vi "Teleop.vi"(10 "Match Info":T1={"Autonomous Elapsed Seconds"=0.0, "TeleOp Elapsed Seconds"=0.0, "Disabled Elapsed Seconds"=0.0, "Visited Autonomous"=FALSE, "Visited TeleOp"=FALSE, "Visited Disabled"=FALSE, "Autonomous Settings"={"Autonomous Style"=enum."Independent", "VI Refnum"=refnum}}, 11 "Call Context":T2) -> ()   [LabVIEW 2015]
doc: "This VI is called for each TeleOp packet received from the DS where the robot is not disabled. It is often used to read from the joysticks and update I/O or to update setpoints for timed control loops. It should complete and return within 20 milliseconds or it may miss DS packets."
uses:
  <vilib>/Rock Robotics/WPI/DriverStation/WPI_DriverStationDerivedRobotMode.ctl
  <vilib>/Rock Robotics/WPI/DriverStation/WPI_DriverStationMatch Info.ctl
  <vilib>/Rock Robotics/WPI/Utilities/WPI_GetSetVariantRefNum.vi
  Robot Global Data.vi
  <vilib>/Rock Robotics/Network Tables/SD Write Number.vi
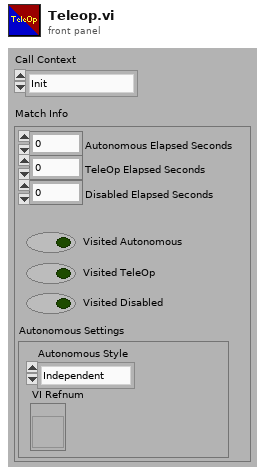
[diagram p1: front panel]
types:
  T1 = typedef "WPI_DriverStationMatch Info.ctl" = cluster{"Autonomous Elapsed Seconds":dbl, "TeleOp Elapsed Seconds":dbl, "Disabled Elapsed Seconds":dbl, "Visited Autonomous":bool, "Visited TeleOp":bool, "Visited Disabled":bool, "Autonomous Settings":cluster{"Autonomous Style":enum16{"Iterative", "Independent"}, "VI Refnum":refnum<vi>}}
  T2 = typedef "WPI_DriverStationDerivedRobotMode.ctl" = enum16{"Init", "Execute", "Stop"}
  T3 = typedef "WPI_RobotDriveDevRef.ctl" = cluster{"DevStatus":errorcluster, "Motors[]":T4[], "Square Inputs":bool, "Max Output":dbl}
  T4 = typedef "WPI_MotorControlDeviceRef.ctl" = cluster{"DeviceStatus":errorcluster, "Type":T5, "PWM":cluster{"PWM Channel":T6, "DeadBand":T7}, "CAN":cluster{"Device Number":u8, "Control Mode":T8, "Semaphore":T9, "Max Vout":dbl, "TalonSRX Control Mode":T10}, "Invert":bool}
  T5 = typedef "WPI_MotorControlType.ctl" = enum16{"PWM", "CAN", "CANTalonSRX"}
  T6 = typedef "FPGA_DIOPWMChannel.ctl" = enum8{"PWM 0", "PWM 1", "PWM 2", "PWM 3", "PWM 4", "PWM 5", "PWM 6", "PWM 7", "PWM 8", "PWM 9", "PWM MXP 0", "PWM MXP 1", "PWM MXP 2", "PWM MXP 3", "PWM MXP 4", "PWM MXP 5", "PWM MXP 6", "PWM MXP 7", "PWM MXP 8", "PWM MXP 9", "Invalid"}
  T7 = typedef "WPI_PWMDeadband.ctl" = cluster{"Name":string, "maxPositivePwm":i32, "minPositivePwm":i32, "centerPwm":i32, "maxNegativePwm":i32, "minNegativePwm":i32, "angularRange":u16}
  T8 = typedef "WPI_CANJaguar_ControlMode.ctl" = enum8{"Percent VBus", "Current", "Speed", "Position", "Voltage"}
  T9 = typedef "Semaphore RefNum" = refnum<k1>
  T10 = typedef "WPI_CANTalonSRX_APIControlMode.ctl" = enum8{"Percent VBus", "Speed", "Position", "Slave", "Unchanged / Invalid", "Voltage Compensation", "Current", "Motion Profile"}
  T11 = typedef "WPI_CANTalonSRX_GlobalStatus.ctl" = cluster{"Applied Throttle":dbl, "Module Enabled":bool, "CAN Error":errorcluster, "Closed Loop Error":dbl, "Forward Limit Switch Closed":bool, "Reverse Limit Switch Closed":bool, "Sensor Position":dbl, "Sensor Velocity":dbl, "Current":dbl, "Sticky Fault - Over Temp":bool, "Sticky Fault - Under Voltage":bool, "Sticky Fault - Forward Limit":bool, "Sticky Fault - Reverse Limit":bool, "Sticky Fault - Forward Soft Limit":bool, "Sticky Fault - Reverse Soft Limit":bool, "Brake is Enabled":bool, "Encoder Position":dbl, "Encoder Velocity":dbl, "Encoder Index Count":dbl, "Encoder A Pin State":bool, "Encoder B Pin State":bool, "Encoder Index Pin State":bool, "Analog In":dbl, "Analog In Velocity":dbl, "Temperature (C)":dbl, "Battery Voltage":dbl, "Control 5 Is Supported":bool, "Current Profile Slot Select":dbl, "Pos Div 8":bool, "Vel Div 4":bool, "Pulse Width Position":i32, "Pulse Width Velocity":i32, "Pulse Width Rise To Rise (us)":i32, "Pulse Width Rise To Fall (us)":i32, "Mot Prof Active Is Under Run":bool, "Mot Prof Active Has Under Run":bool, "Mot Prof Active Is Last":bool, "Mot Prof Active Velocity Only":bool, "Mot Prof Active Is Valid":bool, "Mot Prof Buffer Is Full":bool, "Mot Prof Active Profile Slot Select":i32, "Mot Prof NextID":i32, "Mot Prof Count":i32, "Mot Prof Active Velocity":dbl, "Mot Prof Active Position":dbl, "Mot Prof Output Enable":i32}
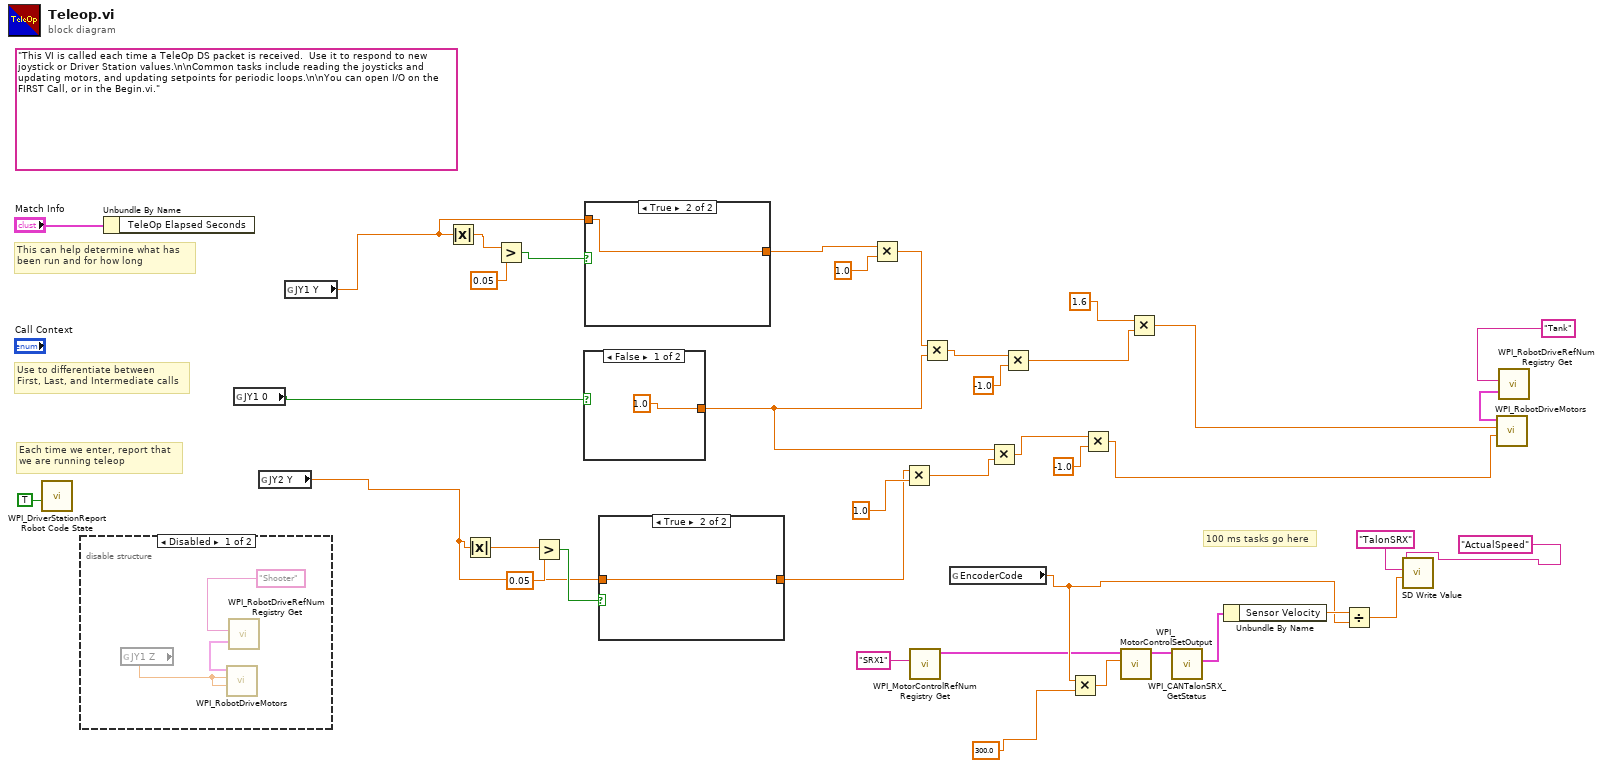
[diagram p0: block diagram]
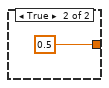
[diagram p3: hidden frame]
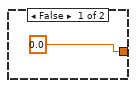
[diagram p4: hidden frame]
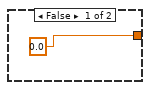
[diagram p5: hidden frame]
diagram:
  (unwired) "This VI is called each time a TeleOp DS packet is received.  Use it to respond to new joystick or Driver Station values.\n\nCommon tasks include reading the joysticks and updating motors, and updating setpoints for periodic loops.\n\nYou can open I/O on the FIRST Call, or in the Begin.vi."
  # "100 ms tasks go here"
  # "Each time we enter, report that\nwe are running teleop"
  # "Use to differentiate between\nFirst, Last, and Intermediate calls"
  # "This can help determine what has\nbeen run and for how long"
  n1 = call <vilib>:"WPI_DriverStationReport Robot Code State.vi"("TeleOp"=TRUE ("Autonomous")) -> ()  [unwired: 10 in, 1 out]
  n2 = disable-structure shown="Disabled" {
    frame Disabled {
      n3 = global read "Robot Global Data.vi" "JY1 Z"() -> (w40:dbl)
      n4 = call <vilib>:"WPI_RobotDriveRefNum Registry Get.vi"("refnum name"="Shooter") -> ("RobotDriveDevRef"=w41:T3)  [unwired: 1 in, 9 out]
      n5 = call <vilib>:"WPI_RobotDriveMotors.vi"("RightSpeed"=w40, "LeftSpeed"=w40, "RobotDriveDevRef"=w41) -> ()  [unwired: 6 in, 3 out]
    }
    frame Enabled {
    }
  }
  n6 = Unbundle By Name("Match Info") -> ()  [unwired: 1 out]
  n7 = global read "Robot Global Data.vi" "JY1 0"() -> (w12:bool)
  n8 = global read "Robot Global Data.vi" "JY2 Y"() -> (w13:dbl)
  n9 = global read "Robot Global Data.vi" "JY1 Y"() -> (w14:dbl)
  n10 = Absolute Value(x=w14) -> (abs(x)=w19:dbl)
  n11 = Absolute Value(x=w13) -> (abs(x)=w18:dbl)
  n12 = Greater?(x=w19, y=0.05) -> (0:w37:bool)
  n13 = Greater?(x=w18, y=0.05) -> (0:w35:bool)
  n14 = case shown="False" w12 {
    tunnel: [1.0 0.5] -> w26
    frame False {
    }
    frame True {
    }
  }
  n15 = case shown="True" w37 {
    tunnel: [0.0 w46] -> w31
    tunnel: w14 -> [_ w46]
    frame False {
    }
    frame True {
    }
  }
  n16 = case shown="True" w35 {
    tunnel: [0.0 w48] -> w30
    tunnel: w13 -> [_ _]
    tunnel: w13 -> [_ w48]
    frame False {
    }
    frame True {
    }
  }
  n17 = Multiply(x=w31, y=1.0) -> (x*y=w27:dbl)
  n18 = Multiply(x=w30, y=1.0) -> (x*y=w25:dbl)
  n19 = call <vilib>:"WPI_MotorControlRefNum Registry Get.vi"("refnum name"="SRX1") -> ("MotorControlDevRef"=w5:T4)  [unwired: 9 in, 1 out]
  n20 = Multiply(x=w27, y=w26) -> (x*y=w24:dbl)
  n21 = global read "Robot Global Data.vi" "EncoderCode"() -> (w7:dbl)
  n22 = Multiply(x=w26, y=w25) -> (x*y=w20:dbl)
  n23 = Multiply(x=w24, y=-1.0) -> (x*y=w16:dbl)
  n24 = Multiply(x=w7, y=300.0) -> (x*y=w8:dbl)
  n25 = Multiply(x=w20, y=-1.0) -> (x*y=w21:dbl)
  n26 = call <vilib>:"WPI_MotorControlSetOutput.vi"("Output"=w8, "MotorControlDevRef"=w5) -> ("MotorControlDevRef"=w11:T4)  [unwired: 7 in, 2 out]
  n27 = Multiply(x=1.6, y=w16) -> (x*y=w15:dbl)
  n28 = call <vilib>:"WPI_CANTalonSRX_GetStatus.vi"("CAN Talon SRX Ref"=w11) -> ("Talon SRX Status"=w10:T11)  [unwired: 8 in, 2 out]
  n29 = Unbundle By Name(w10) -> ("Sensor Velocity"=w9:dbl)
  n30 = Divide(x=w9, y=w7) -> (x/y=w2:dbl)
  n31 = call-poly <vilib>:"SD Write Value.vi"("Numeric"=w2, "Table Prefix"="TalonSRX", "Name"="ActualSpeed") -> ()  [unwired: 7 in, 2 out]
  n32 = call <vilib>:"WPI_RobotDriveRefNum Registry Get.vi"("refnum name"="Tank") -> ("RobotDriveDevRef"=w28:T3)  [unwired: 1 in, 9 out]
  n33 = call <vilib>:"WPI_RobotDriveMotors.vi"("RightSpeed"=w21, "LeftSpeed"=w15, "RobotDriveDevRef"=w28) -> ()  [unwired: 6 in, 3 out]
